vi "Rename Plugin Main VI.vi"(0 "configuration":T1, 5 "Plugin Library Path":path, 11 "error in":errorcluster) -> (4 "Plugin Main VI Path":path, 15 "error out":errorcluster)   [LabVIEW 2021, in "InstrumentStudio Plug-In Editor.lvlib"]
uses:
  InstrumentStudio Plug-In Editor.lvlib
  Data Holder.ctl
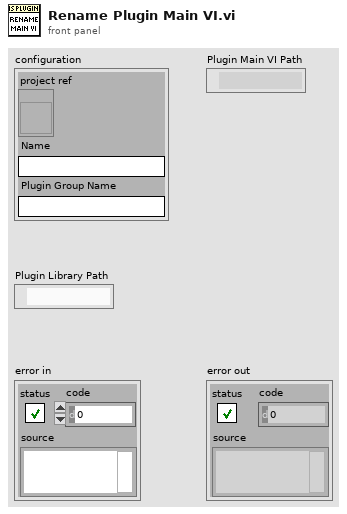
[diagram p1: front panel]
types:
  T1 = typedef "InstrumentStudio Plug-In Editor.lvlib/Data Holder.ctl" = cluster{"project ref":refnum<vi>, "Name":string, "Plugin Group Name":string}
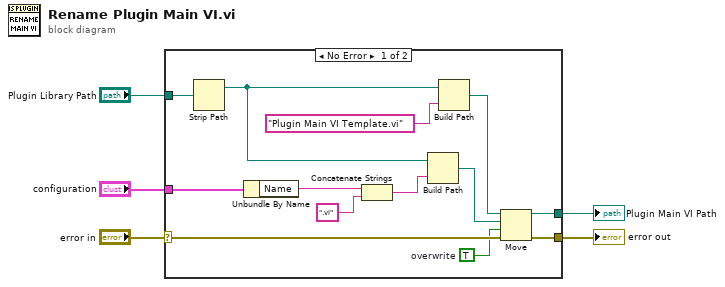
[diagram p0: block diagram]
diagram:
  n1 = case shown="No Error" "error in" {
    selector: "error in" -> [w16 w19]
    tunnel: "Plugin Library Path" -> [w10 _]
    tunnel: [w14 w19] -> w3
    tunnel: [w13 _] -> w2
    tunnel: "configuration" -> [w6 _]
    frame No Error {
      w15 = TRUE  # overwrite
      n2 = Strip Path(path=w10) -> (stripped path=w7:path)  [unwired: 1 out]
      n3 = Unbundle By Name(w6) -> ("Name"=w12:string)
      n4 = Concatenate Strings(w12, ".vi" ("string")) -> (w9:string)
      n5 = Build Path(base path=w7, name or relative path=w9) -> (appended path=w17:path)
      n6 = Build Path(base path=w7, name or relative path="Plugin Main VI Template.vi" ("string")) -> (appended path=w18:path)
      n7 = Move(source path=w18, error in=w16, 9:w15, 10:w17) -> (error out=w14:errorcluster, 3:w13:path)  [unwired: 1 in, 1 out]
    }
    frame Error {
    }
  }
  "error out" <- w3
  "Plugin Main VI Path" <- w2
